vi "Get JSON Value.vi"(8 "error in":errorcluster, 9 "Offset":i32, 10 "$Path or Item Name":string, 11 "JSON in":string) -> (0 "error out":errorcluster, 1 "Found":bool, 3 "Value":string, 4 "Item offset":i32)   [LabVIEW 2020]
uses:
  41463e57-fe3d-40f2-89f5-c7eb17ea6cd4.vi
  <vilib>/JDP Science/JSONtext/Find Item.vi
  <vilib>/JDP Science/JSONtext/String Subset.vi
  <vilib>/JDP Science/JSONtext/Parsing/Parse Full Path or Item Name.vi
  <vilib>/JDP Science/JSONtext/Next JSON Value.vi
  <vilib>/JDP Science/JSONtext/support/Error Cluster From Code.vi
  <vilib>/JDP Science/JSONtext/Offset/Find Item Locations by Path.vi
  <vilib>/JDP Science/JSONtext/JSON text to Variant.vi
  <vilib>/JDP Science/JSONtext/LVClass Serializer/JSONtext LVClass Serializer.lvclass
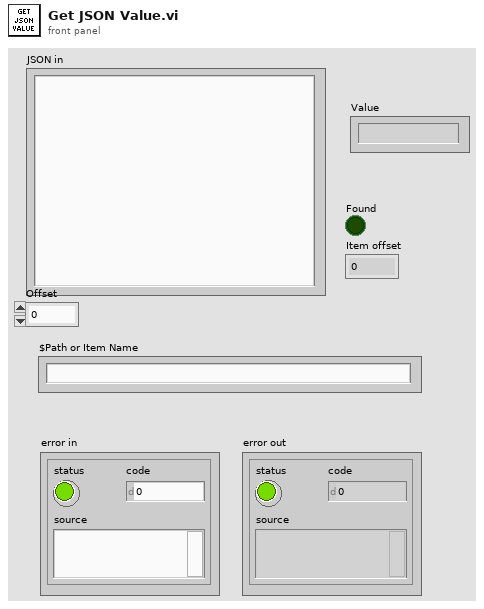
[diagram p1: front panel]
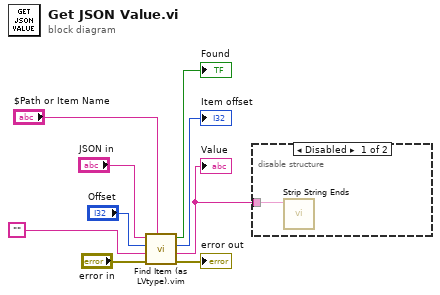
[diagram p0: block diagram]
diagram:
  n1 = call "Find Item (as LVtype).vim"("$Path or Item Name"="$Path or Item Name", "error in (no error)"="error in", "Data Type and Default Value"="", "Offset"="Offset", "JSON"="JSON in") -> ("error out"=→"error out":errorcluster, "Data"=w9:string, "Item offset"=→"Item offset":i32, "Found"=→"Found":bool)  [unwired: 3 in]
  "Value" <- w9
  n2 = disable-structure shown="Disabled" {
    disable-tunnel: w9 -> [w10 _]
    frame Disabled {
      n3 = call "Strip String Ends.vi"("String in"=w10) -> ()  [unwired: 10 in, 1 out]
    }
    frame Enabled {
    }
  }
